vi "actionXML.vi"(8 "error in (no error)":errorcluster, 11 "ScriptEvent in":refnum<class "ScriptEvent.lvclass">) -> (0 "error out":errorcluster, 2 "actionXml":refnum<class "xmlNode.lvclass">, 3 "ScriptEvent out":refnum<class "ScriptEvent.lvclass">)   [LabVIEW 2011, in "Tools.lvlib" / "Scripting.lvlib" / "ScriptEvent.lvclass"]
uses:
  ScriptEvent.lvclass
  xmlNode/xmlNode.lvclass
  ScriptEvent.lvclass/ScriptEvent.ctl
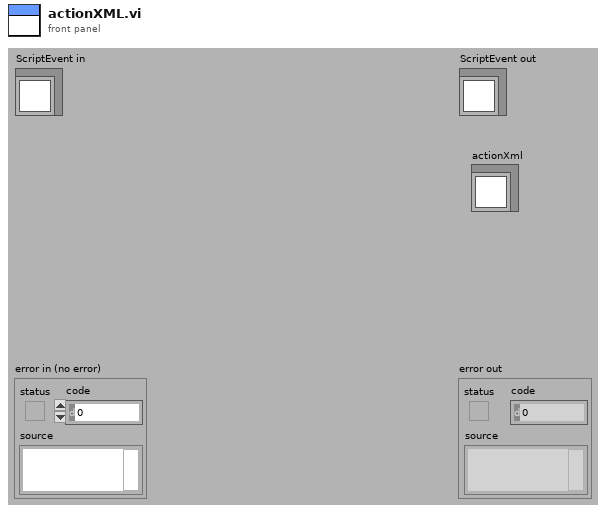
[diagram p1: front panel]
types:
  T1 = enum16{"changeValue", "pulse", "clock", "rampUp", "rampDown", "singleTone", "singleToneRamp", "playFile", "rf", "rfRamp", "delay"}
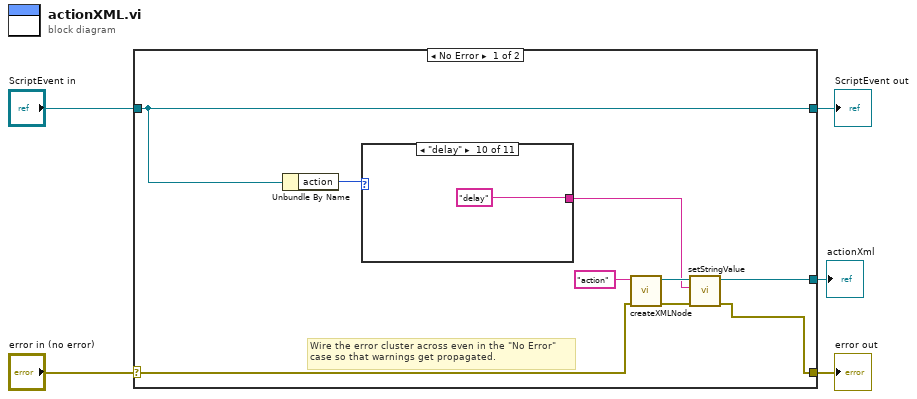
[diagram p0: block diagram]
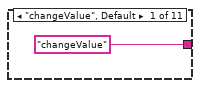
[diagram p2: hidden frame]
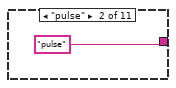
[diagram p3: hidden frame]
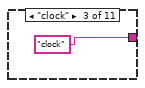
[diagram p4: hidden frame]
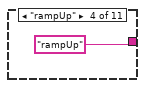
[diagram p5: hidden frame]
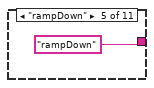
[diagram p6: hidden frame]
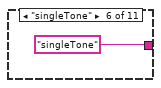
[diagram p7: hidden frame]
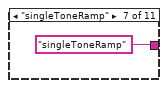
[diagram p8: hidden frame]
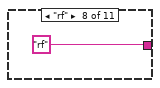
[diagram p9: hidden frame]
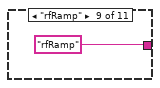
[diagram p10: hidden frame]
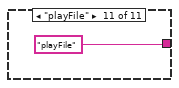
[diagram p11: hidden frame]
diagram:
  n1 = case shown="No Error" "error in (no error)" {
    selector: "error in (no error)" -> [w8 w27]
    tunnel: [w7 w27] -> w4
    tunnel: [w11 w26] -> w2
    tunnel: "ScriptEvent in" -> [w11 w26]
    tunnel: [w6 _] -> w1
    frame No Error {
      # "Wire the error cluster across even in the \"No Error\"\ncase so that warnings get propagated."
      n2 = Unbundle By Name(w11) -> ("action"=w10:T1)
      n3 = case shown="\"delay\"" w10 {
        tunnel: ["changeValue" "pulse" "clock" "rampUp" "rampDown" "singleTone" "singleToneRamp" "rf" "rfRamp" "delay" "playFile"] -> w9
        frame "changeValue", Default {
        }
        frame "pulse" {
        }
        frame "clock" {
        }
        frame "rampUp" {
        }
        frame "rampDown" {
        }
        frame "singleTone" {
        }
        frame "singleToneRamp" {
        }
        frame "rf" {
        }
        frame "rfRamp" {
        }
        frame "delay" {
        }
        frame "playFile" {
        }
      }
      n4 = call "createXMLNode.vi"("error in (no error)"=w8, "name"="action") -> ("error out"=w12:errorcluster, "xmlNode out"=w13:refnum<class "xmlNode.lvclass">)  [unwired: 8 in]
      n5 = call-dynamic "setStringValue.vi"("error in (no error)"=w12, "stringValue"=w9, "xmlNode.lvclass in"=w13) -> ("error out"=w7:errorcluster, "xmlNode.lvclass out"=w6:refnum<class "xmlNode.lvclass">)  [unwired: 7 in]
    }
    frame Error {
    }
  }
  "error out" <- w4
  "ScriptEvent out" <- w2
  "actionXml" <- w1
